vi "Stepper Mover Text Out.vi"(1 "Stepper Mover":T2={"extra wait"=0, "Stepper Value"=1e-09, "Top or Bottom"=enum."Move to Top Position (deg)"} {"extra wait" min=0; "Stepper Value" format="%#.7e"}) -> (0 "Command text":string[][](array[string]))   [LabVIEW 2020]
uses:
  Stepper Mover.ctl
panel:
  out "Est Time (H:M:S)":dbl
  out "Top or Bottom":T1(ring)
  out "String Cluster":T3
  # "Stepper Mover"
  # "(Stepper Mover.vi needs to be open before using this program)"
  # "Value"
  # "seconds"
  # "AND wait extra"
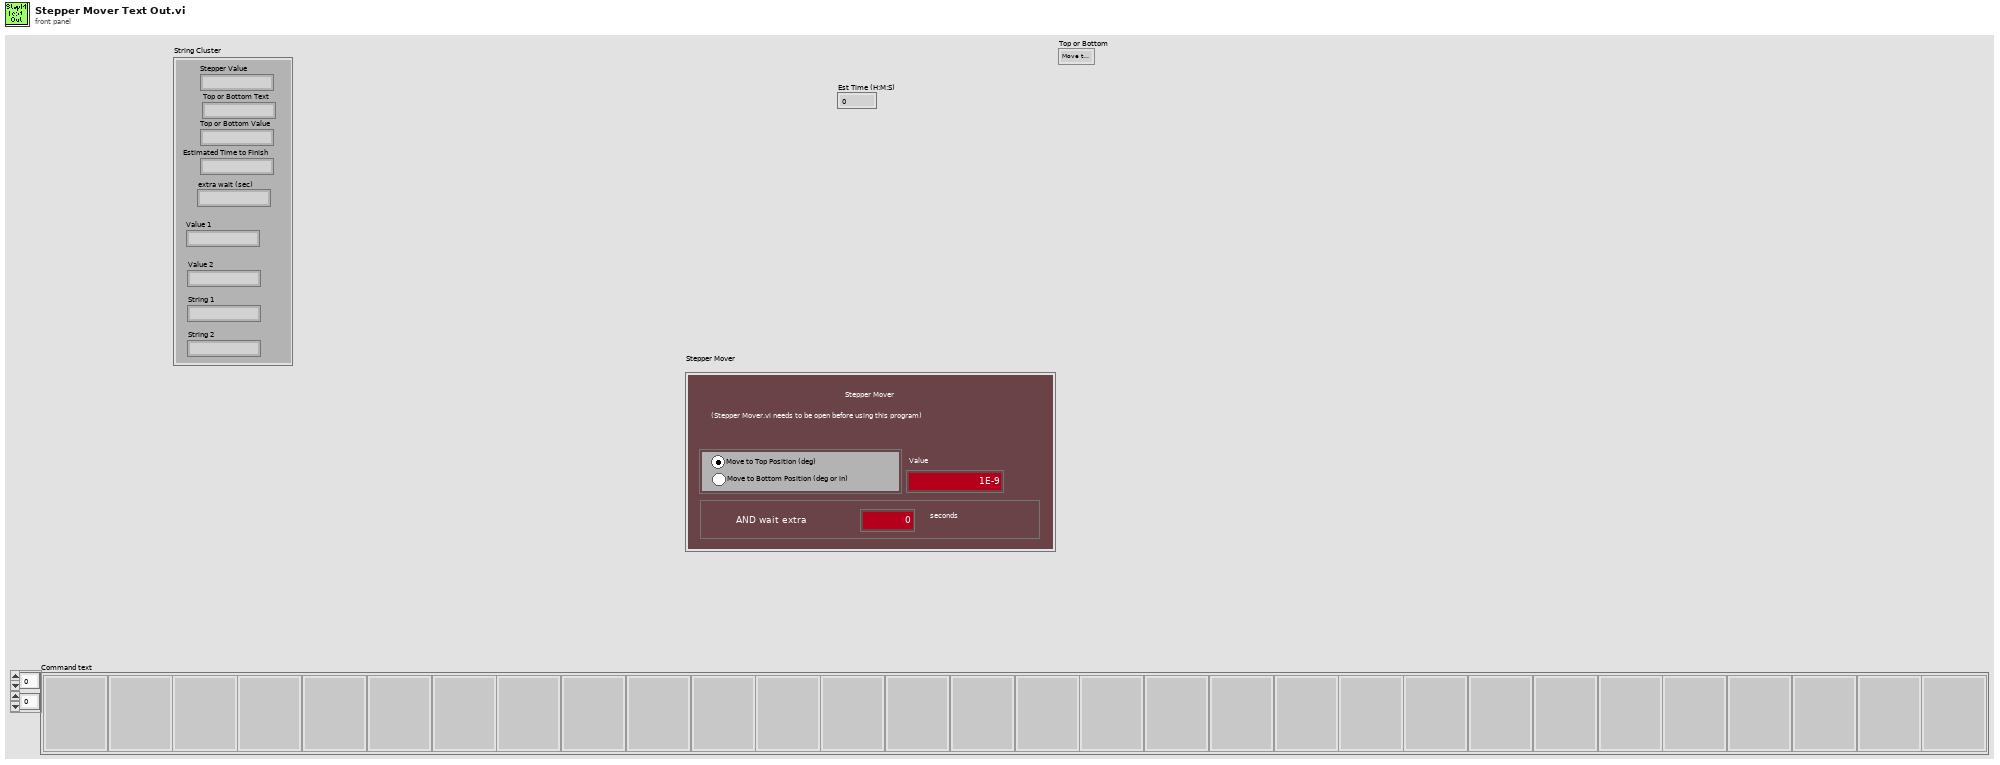
[diagram p1: front panel]
types:
  T1 = enum32{"Move to Top Position (deg)", "Move to Bottom Position (deg or in)"}
  T2 = typedef "Stepper Mover.ctl" = cluster{"extra wait":i32, "Stepper Value":dbl, "Top or Bottom":enum32{"Move to Top Position (deg)", "Move to Bottom Position (deg or in)"}}
  T3 = cluster{"Stepper Value":string, "Top or Bottom Value":string, "Estimated Time to Finish":string, "extra wait (sec)":string, "Top or Bottom Text":string, "Value 1":string, "Value 2":string, "String 1":string, "String 2":string}
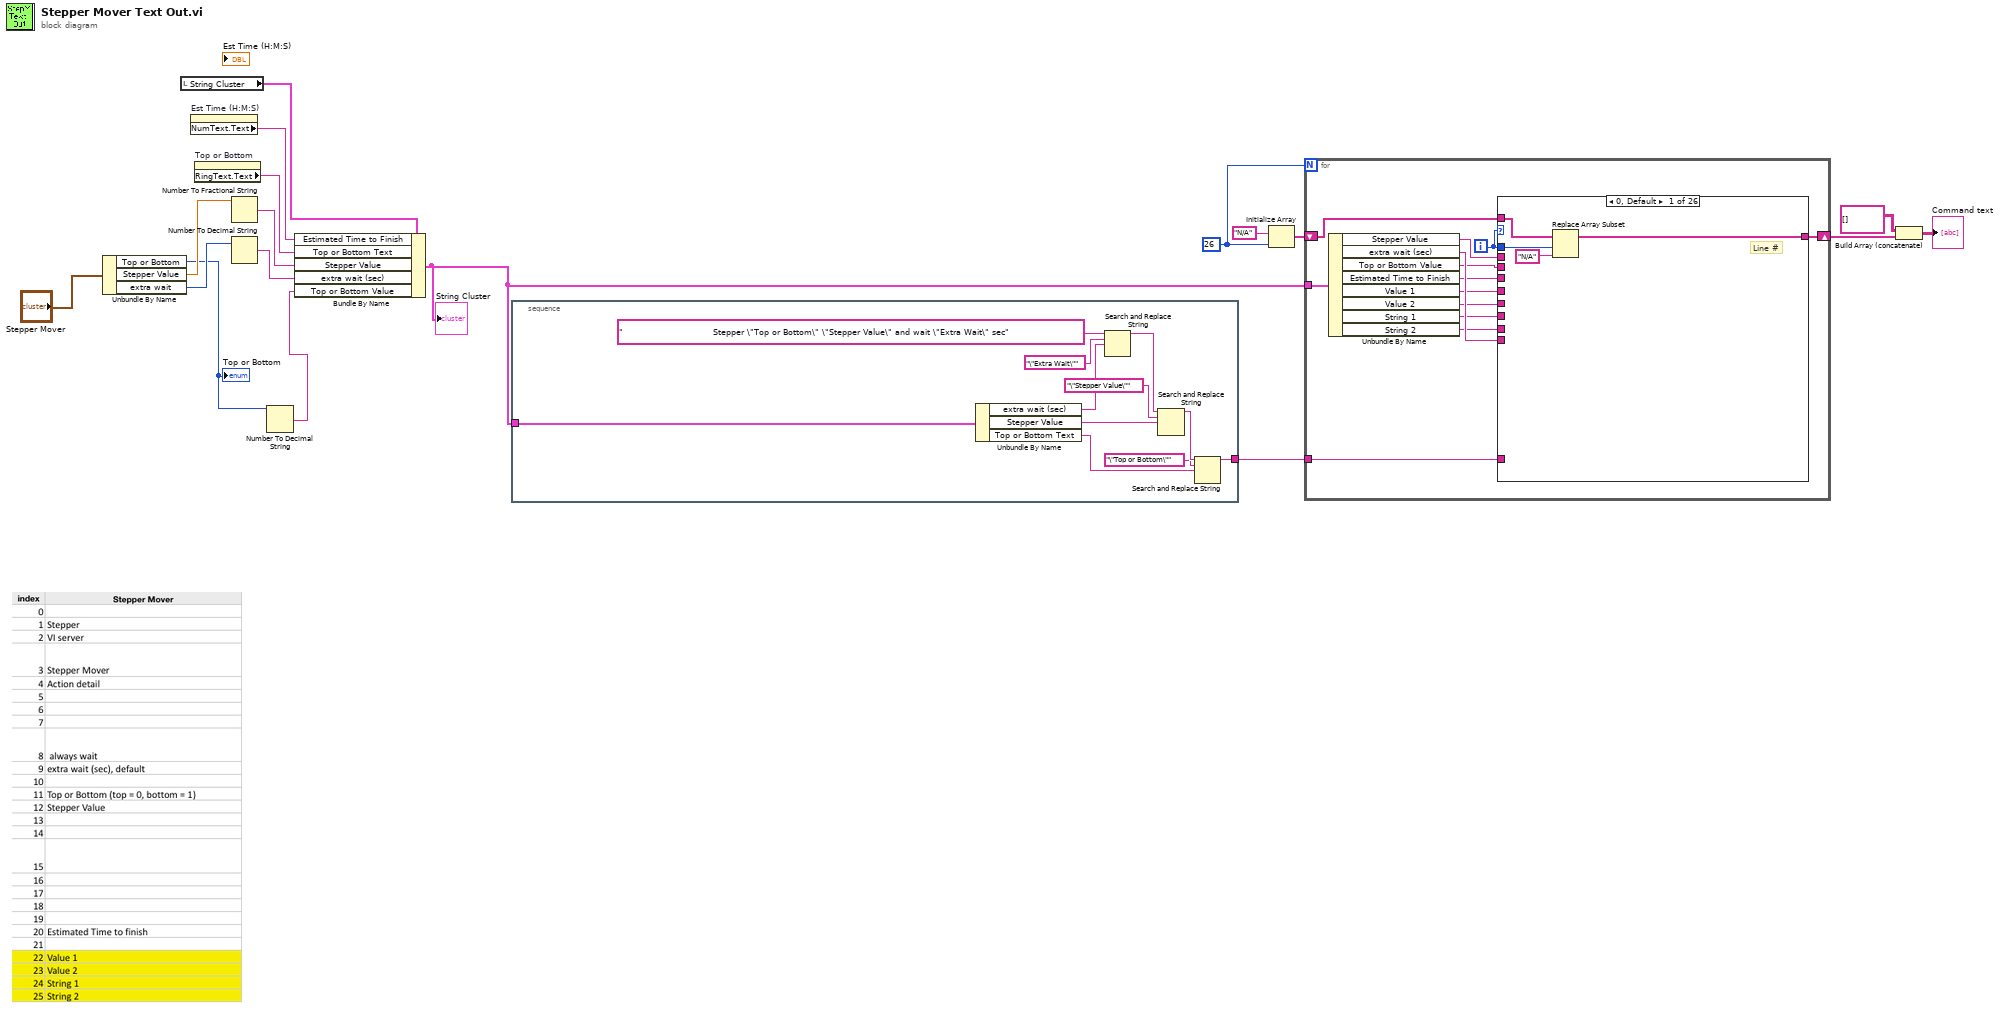
[diagram p0: block diagram]
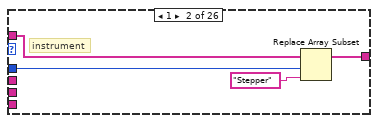
[diagram p2: hidden frame]
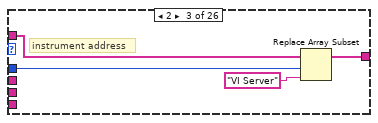
[diagram p3: hidden frame]
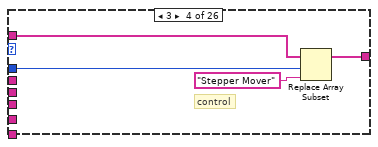
[diagram p4: hidden frame]
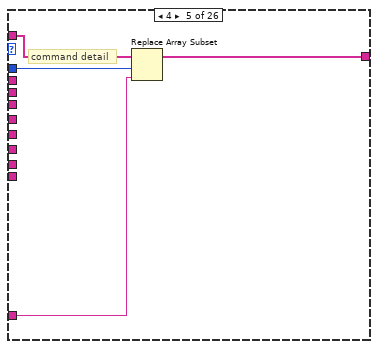
[diagram p5: hidden frame]
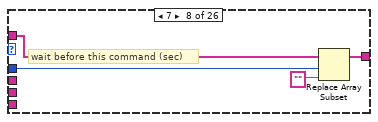
[diagram p8: hidden frame]
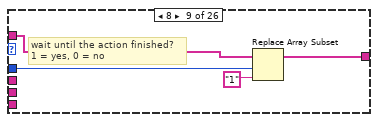
[diagram p9: hidden frame]
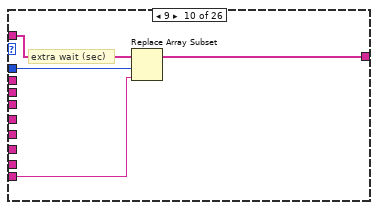
[diagram p10: hidden frame]
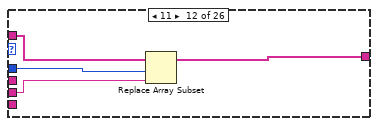
[diagram p12: hidden frame]
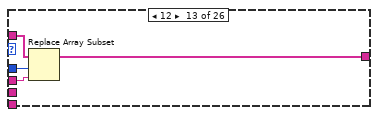
[diagram p13: hidden frame]
diagram:
  w15 = 26
  n1 = Unbundle By Name("Stepper Mover") -> ("Top or Bottom"=w2:T1, "Stepper Value"=w5:dbl, "extra wait"=w8:i32)
  "Top or Bottom" <- w2
  n2 = local read "String Cluster"() -> (w12:T3)
  n3 = property on="Est Time (H:M:S)" class="DigNum (strict)"() -> ("NumText.Text"=w3:string)  [unwired: 2 in, 2 out]
  n4 = property on="Top or Bottom" class="Enum (strict)"() -> ("RingText.Text"=w6:string)  [unwired: 2 in, 2 out]
  n5 = Number To Fractional String(number=w5) -> (F-format string=w4:string)  [unwired: 3 in]
  n6 = Number To Decimal String(number=w8) -> (decimal integer string=w7:string)  [unwired: 1 in]
  n7 = Number To Decimal String(number=w2) -> (decimal integer string=w1:string)  [unwired: 1 in]
  n8 = Bundle By Name(cluster=w12, "Estimated Time to Finish"=w3, "Top or Bottom Text"=w6, "Stepper Value"=w4, "extra wait (sec)"=w7, "Top or Bottom Value"=w1) -> (w10:T3)
  "String Cluster" <- w10
  n9 = stacked-sequence {
    tunnel: [w19] -> w11
    tunnel: w10 -> [w23]
    frame #0 {
      n10 = Unbundle By Name(w23) -> ("extra wait (sec)"=w22:string, "Stepper Value"=w21:string, "Top or Bottom Text"=w20:string)
      n11 = Search and Replace String(input string="                              Stepper \"Top or Bottom\" \"Stepper Value\" and wait \"Extra Wait\" sec", search string="\"Extra Wait\"", replace string=w22) -> (result string=w28:string)  [unwired: 5 in, 3 out]
      n12 = Search and Replace String(input string=w28, search string="\"Stepper Value\"", replace string=w21) -> (result string=w29:string)  [unwired: 5 in, 3 out]
      n13 = Search and Replace String(input string=w29, search string="\"Top or Bottom\"", replace string=w20) -> (result string=w19:string)  [unwired: 5 in, 3 out]
    }
  }
  n14 = Initialize Array("N/A", w15) -> (w14:string[])
  n15 = for {
    N: w15 -> [_]
    shift-right: [w40] -> w13
    shift-left: w14 -> [w41]
    tunnel: w11 -> [w39]
    tunnel: w10 -> [w38]
    i -> [w42]
    n16 = Unbundle By Name(w38) -> ("Stepper Value"=w37:string, "extra wait (sec)"=w36:string, "Top or Bottom Value"=w31:string, "Estimated Time to Finish"=w30:string, "Value 1"=w35:string, "Value 2"=w34:string, "String 1"=w33:string, "String 2"=w32:string)
    n17 = case shown="0, Default" w42 {
      tunnel: w42 -> [w45 w49 w54 w56 w61 _ _ w66 w70 w74 _ w79 w83 _ _ _ _ _ _ _ w94 _ w98 w103 w107 w111]
      tunnel: w41 -> [w46 w48 w53 w57 w62 w63 w64 w68 w72 w76 w77 w80 w85 w86 w87 w88 w89 w90 w91 w92 w96 w97 w100 w105 w109 w112]
      tunnel: [w43 w47 w52 w55 w60 w63 w64 w67 w71 w75 w77 w81 w84 w86 w87 w88 w89 w90 w91 w92 w95 w97 w99 w104 w108 w113] -> w40
      tunnel: w39 -> [_ _ _ _ w59 _ _ _ _ _ _ _ _ _ _ _ _ _ _ _ _ _ _ _ _ _]
      tunnel: w37 -> [_ _ _ _ _ _ _ _ _ _ _ _ w82 _ _ _ _ _ _ _ _ _ _ _ _ _]
      tunnel: w36 -> [_ _ _ _ _ _ _ _ _ w73 _ _ _ _ _ _ _ _ _ _ _ _ _ _ _ _]
      tunnel: w35 -> [_ _ _ _ _ _ _ _ _ _ _ _ _ _ _ _ _ _ _ _ _ _ w101 _ _ _]
      tunnel: w34 -> [_ _ _ _ _ _ _ _ _ _ _ _ _ _ _ _ _ _ _ _ _ _ _ w102 _ _]
      tunnel: w33 -> [_ _ _ _ _ _ _ _ _ _ _ _ _ _ _ _ _ _ _ _ _ _ _ _ w106 _]
      tunnel: w32 -> [_ _ _ _ _ _ _ _ _ _ _ _ _ _ _ _ _ _ _ _ _ _ _ _ _ w110]
      tunnel: w31 -> [_ _ _ _ _ _ _ _ _ _ _ w78 _ _ _ _ _ _ _ _ _ _ _ _ _ _]
      tunnel: w30 -> [_ _ _ _ _ _ _ _ _ _ _ _ _ _ _ _ _ _ _ _ w93 _ _ _ _ _]
      frame 0, Default {
        # "Line #"
        n18 = Replace Array Subset(array=w46, new element="N/A", index=w45) -> (w43:string[])
      }
      frame 1 {
        # "instrument"
        n19 = Replace Array Subset(array=w48, new element="Stepper", index=w49) -> (w47:string[])
      }
      frame 2 {
        # "instrument address"
        n20 = Replace Array Subset(array=w53, new element="VI Server" ("new element/subarray"), index=w54) -> (w52:string[])
      }
      frame 3 {
        # "control"
        n21 = Replace Array Subset(array=w57, new element="Stepper Mover", index=w56) -> (w55:string[])
      }
      frame 4 {
        # "command detail"
        n22 = Replace Array Subset(array=w62, new element=w59, index=w61) -> (w60:string[])
      }
      frame 5 {
        # "in  case 1"
      }
      frame 6 {
        # "in case 2"
      }
      frame 7 {
        # "wait before this command (sec)"
        n23 = Replace Array Subset(array=w68, new element="" ("new element/subarray"), index=w66) -> (w67:string[])
      }
      frame 8 {
        # "wait until the action finished?\n1 = yes, 0 = no"
        n24 = Replace Array Subset(array=w72, new element="1", index=w70) -> (w71:string[])
      }
      frame 9 {
        # "extra wait (sec)"
        n25 = Replace Array Subset(array=w76, new element=w73, index=w74) -> (w75:string[])
      }
      frame 10 {
      }
      frame 11 {
        n26 = Replace Array Subset(array=w80, new element=w78, index=w79) -> (w81:string[])
      }
      frame 12 {
        n27 = Replace Array Subset(array=w85, new element=w82, index=w83) -> (w84:string[])
      }
      frame 13 {
      }
      frame 14 {
      }
      frame 15 {
      }
      frame 16 {
      }
      frame 17 {
      }
      frame 18 {
      }
      frame 19 {
      }
      frame 20 {
        n28 = Replace Array Subset(array=w96, new element=w93, index=w94) -> (w95:string[])
      }
      frame 21 {
      }
      frame 22 {
        n29 = Replace Array Subset(array=w100, new element=w101, index=w98) -> (w99:string[])
      }
      frame 23 {
        n30 = Replace Array Subset(array=w105, new element=w102, index=w103) -> (w104:string[])
      }
      frame 24 {
        n31 = Replace Array Subset(array=w109, new element=w106, index=w107) -> (w108:string[])
      }
      frame 25 {
        n32 = Replace Array Subset(array=w112, new element=w110, index=w111) -> (w113:string[])
      }
    }
  }
  n33 = Build Array (concatenate)(string[][] [], w13) -> (→"Command text":string[][])
